vi "Write Interlock_Enable.vi"(8 "error in":errorcluster, 10 "INTLK_Enable":bool, 11 "36234A in":refnum<class "36234A.lvclass">) -> (0 "error out":errorcluster, 3 "36234A out":refnum<class "36234A.lvclass">)   [LabVIEW 2019, in "36234A.lvlib" / "36234A.lvclass"]
uses:
  Library/36234A.lvclass
  builds/Instruments/PowerSupply.lvlibp/Library/PowerSupply.lvclass
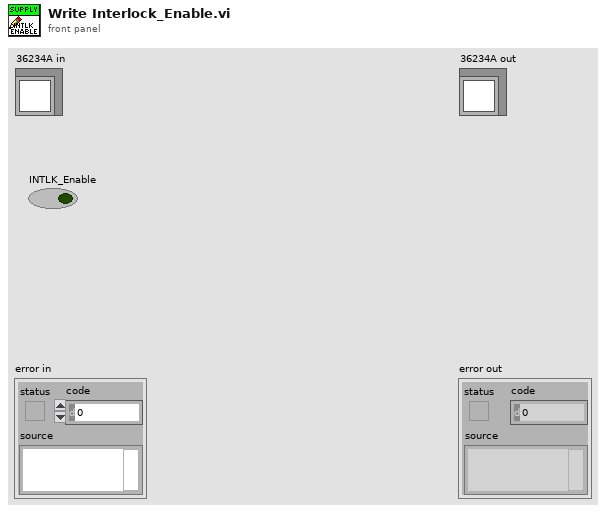
[diagram p1: front panel]
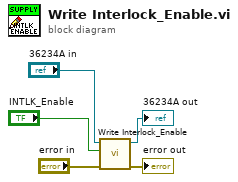
[diagram p0: block diagram]
diagram:
  n1 = call-parent "Write Interlock_Enable.vi"("error in"="error in", "INTLK_Enable"="INTLK_Enable", "PowerSupply in"="36234A in") -> ("error out"=→"error out":errorcluster, "PowerSupply out"=→"36234A out":refnum<class "36234A.lvclass">)  [unwired: 7 in]
